vi "StopSync.vi"(8 "error in (no error)":errorcluster, 11 "NiPxi6682 in":refnum<class "NiPxi6682.lvclass">) -> (0 "error out":errorcluster, 3 "NiPxi6682 out":refnum<class "NiPxi6682.lvclass">)   [LabVIEW 2014, in "SyncPlugins.lvlib" / "NiPxi6682.lvclass"]
uses:
  NiPxi6682.lvclass
  NiPxi6682.lvclass/NiPxi6682.ctl
  SyncPluginBase/SyncPluginBase.lvclass/SyncPluginBase.ctl
  Accessors/Read PgmPPS.vi
  Accessors/Read NiSyncHandle.vi
  Accessors/Read 1PPS.vi
  Accessors/Read DDSHandle.vi
  Accessors/Read clkDiscSession.vi
  SyncPluginBase/Accessors/Write Initiated.vi
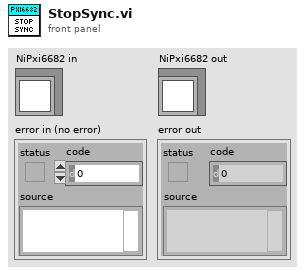
[diagram p1: front panel]
types:
  T1 = typedef "_clkDisc_session.ctl" = variant
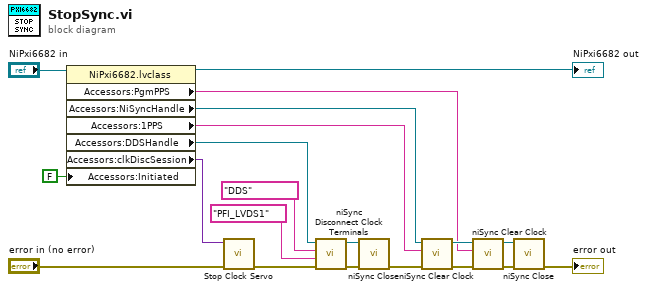
[diagram p0: block diagram]
diagram:
  n1 = property class="NiPxi6682.lvclass"(reference="NiPxi6682 in", "Accessors:Initiated"=FALSE ("Initiated")) -> (reference out=→"NiPxi6682 out":refnum<class "NiPxi6682.lvclass">, "Accessors:PgmPPS"=w7:tag, "Accessors:NiSyncHandle"=w8:refnum<k15>, "Accessors:1PPS"=w9:tag, "Accessors:DDSHandle"=w10:refnum<k15>, "Accessors:clkDiscSession"=w11:T1)  [unwired: 1 in, 1 out]
  n2 = call <userlib>:"Stop Clock Servo.vi"("error (in)"="error in (no error)", "clkDisc session (in)"=w11) -> ("error (out)"=w18:errorcluster)  [unwired: 5 in]
  n3 = call <instrlib>:"niSync Disconnect Clock Terminals.vi"("error in (no error)"=w18, "destination terminal"="PFI_LVDS1", "source terminal"="DDS", "instrument handle"=w10) -> ("error out"=w15:errorcluster, "instrument handle out"=w14:refnum<k15>)  [unwired: 6 in]
  n4 = call <instrlib>:"niSync Close.vi"("error in (no error)"=w15, "instrument handle"=w14) -> ("error out"=w2:errorcluster)  [unwired: 9 in]
  n5 = call <instrlib>:"niSync Clear Clock.vi"("error in (no error)"=w2, "terminal"=w9, "instrument handle"=w8) -> ("error out"=w13:errorcluster, "instrument handle out"=w12:refnum<k15>)  [unwired: 6 in]
  n6 = call <instrlib>:"niSync Clear Clock.vi"("error in (no error)"=w13, "terminal"=w7, "instrument handle"=w12) -> ("error out"=w6:errorcluster, "instrument handle out"=w5:refnum<k15>)  [unwired: 6 in]
  n7 = call <instrlib>:"niSync Close.vi"("error in (no error)"=w6, "instrument handle"=w5) -> ("error out"=→"error out":errorcluster)  [unwired: 9 in]
